vi "Actor Core.vi"(8 "error in":errorcluster, 11 "Nested in":refnum<class "CONTEO_DIG.lvclass">) -> (0 "error out":errorcluster, 3 "Actor out":refnum<class "Actor.lvclass">)   [LabVIEW 2019, in "CONTEO_DIG.lvlib" / "CONTEO_DIG.lvclass"]
doc: "(<B>Filename</B>: Actor Framework.lvlib:Actor.lvclass:Actor Core.vi)\n\nReceives messages to the actor, reacts to them, and initiates any error handling that may shut the actor down.\n\nDescendant classes may override this VI to append parallel tasks for the actor to complete while it handles messages. Overrides use the Call Parent Method node."
uses:
  CONTEO_DIG.lvclass
  C:/Program Files (x86)/National Instruments/LabVIEW 2019/vi.lib/ActorFramework/Actor/Actor.lvclass
  <vilib>/ActorFramework/Actor/Actor.lvclass
  CONTADOR_CON_LIMITES/CONTADOR_CON_LIMITES/CONTADOR_CON_LIMITES.lvclass
  <vilib>/ActorFramework/Actor/Actor.lvclass/Actor.ctl
  <vilib>/ActorFramework/Message Enqueuer/Message Enqueuer.lvclass/Message Enqueuer.ctl
  CONTEO_DIG.lvclass/CONTEO_DIG.ctl
  CONTADOR_CON_LIMITES/CONTADOR_CON_LIMITES Messages/START_STOP_SEND Msg/START_STOP_SEND Msg.lvclass/START_STOP_SEND Msg.ctl
  CONTADOR_CON_LIMITES/CONTADOR_CON_LIMITES Messages/SOLICITAR_LIMITES Msg/SOLICITAR_LIMITES Msg.lvclass/SOLICITAR_LIMITES Msg.ctl
  <vilib>/ActorFramework/Message Enqueuer/Init from Existing Queue.vi
  <vilib>/ActorFramework/Message Enqueuer/Enqueue.vi
  <vilib>/ActorFramework/Stop Msg/Stop Msg.lvclass
  C:/Program Files (x86)/National Instruments/LabVIEW 2019/vi.lib/ActorFramework/Message/Message.lvclass
  CONTADOR_CON_LIMITES/CONTADOR_CON_LIMITES Messages/START_STOP_SEND Msg/START_STOP_SEND Msg.lvclass
  CONTADOR_CON_LIMITES/CONTADOR_CON_LIMITES Messages/SOLICITAR_LIMITES Msg/SOLICITAR_LIMITES Msg.lvclass
  <vilib>/ActorFramework/Message Priority Queue/Priority Enqueue.vi
  <vilib>/ActorFramework/Message Enqueuer/Message Enqueuer.lvclass
panel:
  in  "LÍMITES":T1
  in  "EXIT":bool
  in  "stop":bool
  in  "START":bool
  out "CONTEO":bool[](array[boolean])
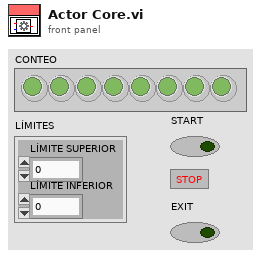
[diagram p1: front panel]
types:
  T1 = cluster{"LÍMITE SUPERIOR":dbl, "LÍMITE INFERIOR":dbl}
  T2 = cluster{"Stop":refnum<user-event>, "CONTEO":refnum<user-event>}
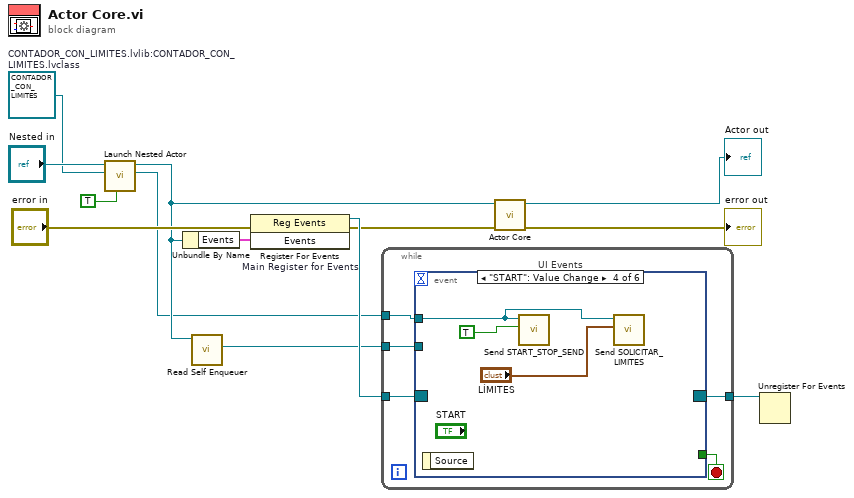
[diagram p0: block diagram]
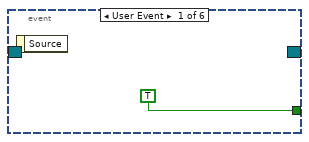
[diagram p2: hidden frame]
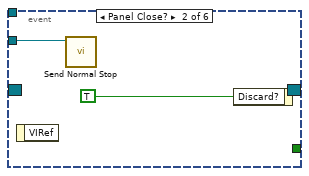
[diagram p3: hidden frame]
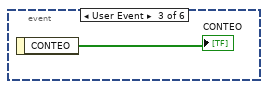
[diagram p4: hidden frame]
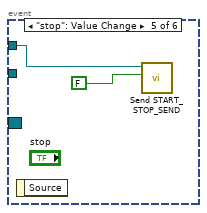
[diagram p5: hidden frame]
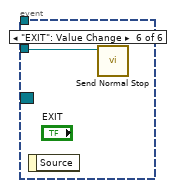
[diagram p6: hidden frame]
diagram:
  w3 = refnum<class "CONTADOR_CON_LIMITES.lvclass"> refnum  # CONTADOR_CON_LIMITES.lvlib:CONTADOR_CON_LIMITES.lvclass
  n1 = call <vilib>:"Launch Nested Actor.vi"("Open Actor Core front panel? (F)"=TRUE, "Nested Actor"=w3, "Caller Actor in"="Nested in") -> ("Nested Actor's Enqueuer"=w2:refnum<class "Message Enqueuer.lvclass">, "Caller Actor out"=w4:refnum<class "CONTEO_DIG.lvclass">)  [unwired: 6 in, 1 out]
  n2 = Unbundle By Name(w4) -> ("Events"=w10:T2)
  n3 = call <vilib>:"Read Self Enqueuer.vi"("Actor"=w4) -> ("Self Enqueuer"=w8:refnum<class "Message Enqueuer.lvclass">)  [unwired: 10 in]
  n4 = register-events "Main Register for Events"(error in="error in", w10) -> (reference out=w11:refnum<event-registration>, error out=w6:errorcluster)  [unwired: 1 in]
  n5 = while {
    tunnel: w11 -> [w18]
    tunnel: [w16] -> w9
    tunnel: w8 -> [w15]
    tunnel: w2 -> [w14]
    stop <- w17 stop-if-true
    n6 = event "UI Events" shown="[3] \"START\": Value Change" {
      selector: w18 -> [_ _ _ _ _ _]
      dyn-events: [_ _ _ _ _ _] -> w16
      timeout: _ -> [_ _ _ _ _ _]
      tunnel: [TRUE _ _ _ _ _] -> w17
      tunnel: w15 -> [_ w20 _ _ _ w28]
      tunnel: w14 -> [_ _ _ w23 w27 _]
      event User Event {
        n7 = event-data() -> ()  [unwired: 1 in, 1 out]
      }
      event Panel Close? {
        n8 = event-data() -> ()  [unwired: 1 in, 1 out]
        n9 = call <vilib>:"Send Normal Stop.vi"("Message Enqueuer"=w20) -> ()  [unwired: 10 in, 1 out]
        n10 = event-data("Discard?"=TRUE) -> ()  [unwired: 1 in, 1 out]
      }
      event User Event {
        n11 = event-data() -> ("CONTEO"=→"CONTEO":bool[])  [unwired: 1 in]
      }
      event "START": Value Change {
        n12 = event-data() -> ()  [unwired: 1 in, 1 out]
        n13 = call "Send START_STOP_SEND.vi"("START/STOP"=TRUE, "Message Enqueuer"=w23) -> ()  [unwired: 8 in, 2 out]
        n14 = call "Send SOLICITAR_LIMITES.vi"("LÍMITES"="LÍMITES", "Message Enqueuer"=w23) -> ()  [unwired: 8 in, 2 out]
      }
      event "stop": Value Change {
        n15 = event-data() -> ()  [unwired: 1 in, 1 out]
        n16 = call "Send START_STOP_SEND.vi"("START/STOP"=FALSE, "Message Enqueuer"=w27) -> ()  [unwired: 8 in, 2 out]
      }
      event "EXIT": Value Change {
        n17 = event-data() -> ()  [unwired: 1 in, 1 out]
        n18 = call <vilib>:"Send Normal Stop.vi"("Message Enqueuer"=w28) -> ()  [unwired: 10 in, 1 out]
      }
    }
  }
  n19 = call-parent "Actor Core.vi"("error in"=w6, "Actor in"=w4) -> ("error out"=→"error out":errorcluster, "Actor out"=→"Actor out":refnum<class "Actor.lvclass">)  [unwired: 8 in]
  n20 = Unregister For Events(event registration refnum=w9) -> ()  [unwired: 1 in, 1 out]
